vi "Validate Incoming Packet.vi"(8 "error in (no error)":errorcluster, 10 "ControlPacket":refnum<class "ControlPacket.lvclass">, 11 "Session in":refnum<class "Session.lvclass">) -> (0 "error out":errorcluster, 2 "ControlPacket out":refnum<class "ControlPacket.lvclass">, 3 "Session out":refnum<class "Session.lvclass">)   [LabVIEW 2013, in "MQTT Base.lvlib" / "Session.lvclass"]
uses:
  Session.lvclass
  <vilib>/LabVIEW Open Source Project/MQTT Control Packets/Control Packets/ControlPacket/ControlPacket.lvclass
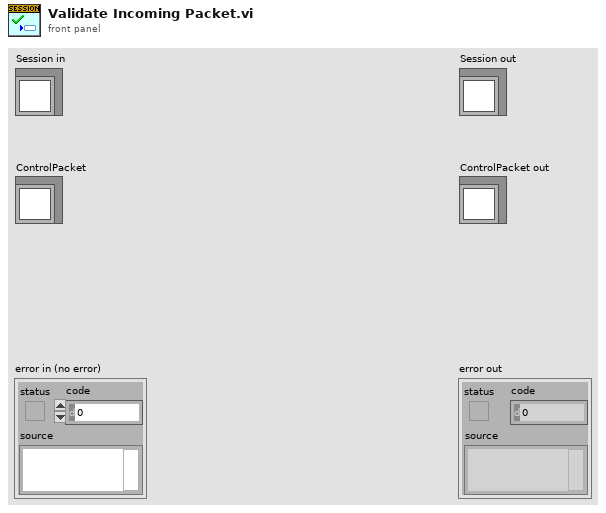
[diagram p1: front panel]
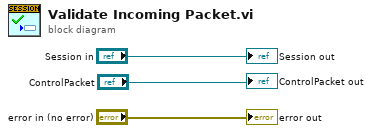
[diagram p0: block diagram]
diagram:
  "error out" <- "error in (no error)"
  "Session out" <- "Session in"
  "ControlPacket out" <- "ControlPacket"
